vi "Bubble sort.vi"(0 "Unsorted Array":dbl[](array[numeric])) -> (4 "Sorted Array":dbl[](array[numeric]))   [LabVIEW 2014]
doc: "Bubble sort."
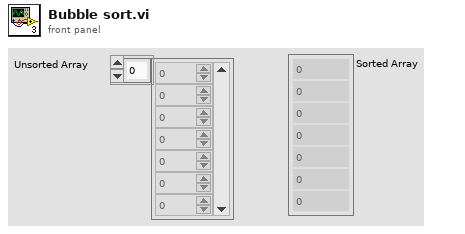
[diagram p1: front panel]
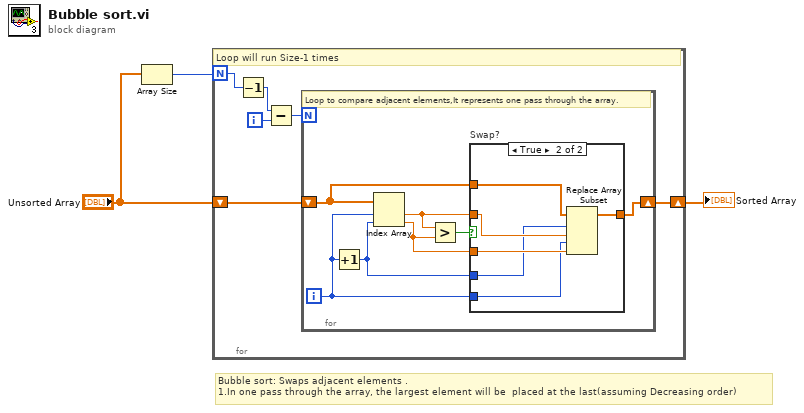
[diagram p0: block diagram]
diagram:
  # "Bubble sort: Swaps adjacent elements .\n1.In one pass through the array, the largest element will be  placed at the last(assuming Decreasing order)"
  n1 = Array Size(array="Unsorted Array") -> (size(s)=w1:i32)
  n2 = for {
    N: w1 -> [w9]
    shift-right: [w4] -> w2
    shift-left: "Unsorted Array" -> [w5]
    i -> [w7]
    # "Loop will run Size-1 times"
    n3 = Decrement(x=w9) -> (x-1=w6:i32)
    n4 = Subtract(x=w6, y=w7) -> (x-y=w8:i32)
    n5 = for {
      N: w8 -> [_]
      shift-right: [w10] -> w4
      shift-left: w5 -> [w15]
      i -> [w13]
      # "Loop to compare adjacent elements,It represents one pass through the array."
      n6 = Increment(x=w13) -> (x+1=w11:i32)
      n7 = Index Array(array=w15, index #1=w13, index #2=w11) -> (element #1=w12:dbl, element #2=w14:dbl)
      n8 = Greater?(x=w12, y=w14) -> (0:w16:bool)
      n9 = case "Swap?" shown="True" w16 {
        tunnel: [w17 w23] -> w10
        tunnel: w15 -> [w17 w22]
        tunnel: w14 -> [_ w21]
        tunnel: w13 -> [_ w20]
        tunnel: w12 -> [_ w19]
        tunnel: w11 -> [_ w18]
        frame False {
          # "Dont swap"
        }
        frame True {
          # "a>b,swap them"
          n10 = Replace Array Subset(array=w22, new element #1=w19, index #1=w18, new element #2=w21, index #2=w20) -> (w23:dbl[])
        }
      }
    }
  }
  "Sorted Array" <- w2
